vi "Tester by yuval.vi"() -> ()   [LabVIEW 2015]
uses:
  source/controls/Treatment Parameters.ctl
  source/controls/Results.ctl
  <vilib>/vision/Image Controls.llb/IMAQ Image.ctl
  <vilib>/vision/driver/NI_Vision_Acquisition_Software.lvlib
  <resource>/objmgr/imaqdx.rc
  <vilib>/vision/NI_Vision_Development_Module.lvlib
panel:
  out "Image Out":T1
  out "Sclera Score":dbl
  out "Results Out":T2={"Center X"=500, "Center Y"=500, "Radius X"=1, "Radius Y"=1, "Circle Match Score"=0, "Sclera Score"=0.0, "Circle Fit Strength"=0, "Circle Match Threshold"=0}
  in  "Camera Name":refnum<k21> caption="IMAQdx Session"
  in  "Video Modes":i32(listbox)
  in  "Stop":bool
  out "Buffer Number":u32
  out "Frame Rate":dbl(knob) scale=0.0..100.0
  out "adjust limbus time":u32
  out "sclera plane time":u32
  in  "Treatment":T3={"Location"=25.0, "Width"=10.0, "Search"=enum."Lower"}
  out "error out":errorcluster
  out "Output Image":T1(plugin-control)
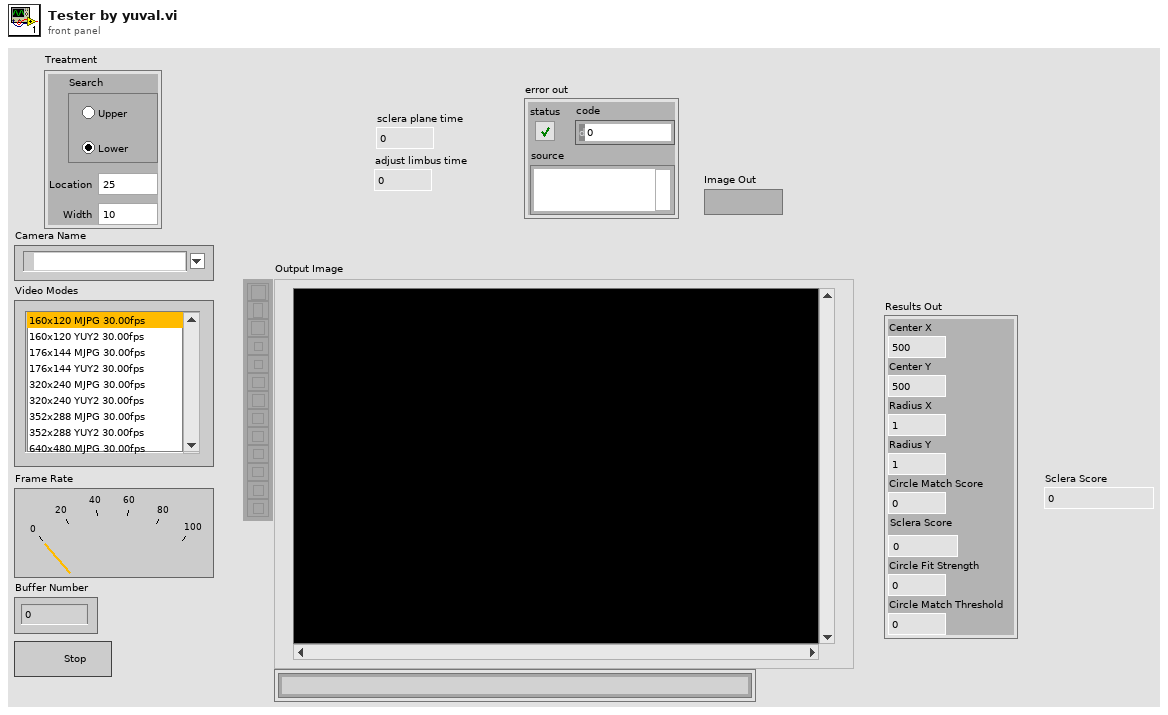
[diagram p1: front panel]
types:
  T1 = typedef "IMAQ Image.ctl" = refnum<image>
  T2 = typedef "Results.ctl" = cluster{"Center X":i32, "Center Y":i32, "Radius X":i32, "Radius Y":i32, "Circle Match Score":i32, "Sclera Score":dbl, "Circle Fit Strength":i32, "Circle Match Threshold":i32}
  T3 = typedef "Treatment Parameters.ctl" = cluster{"Location":dbl, "Width":dbl, "Search":enum32{"Upper", "Lower"}}
  T4 = typedef "IMAQdx.ctl" = refnum<k21>
  T5 = typedef "Images.ctl" = cluster{"Input":T1, "Output":T1, "BufferGray1":T1, "BufferGray2":T1, "TemplatesDown":T1[], "TemplatesUp":T1[], "BufferColor1":T1, "GreenPlane":T1, "ScleraPlane":T1, "RedPlane":T1, "BluePlane":T1}
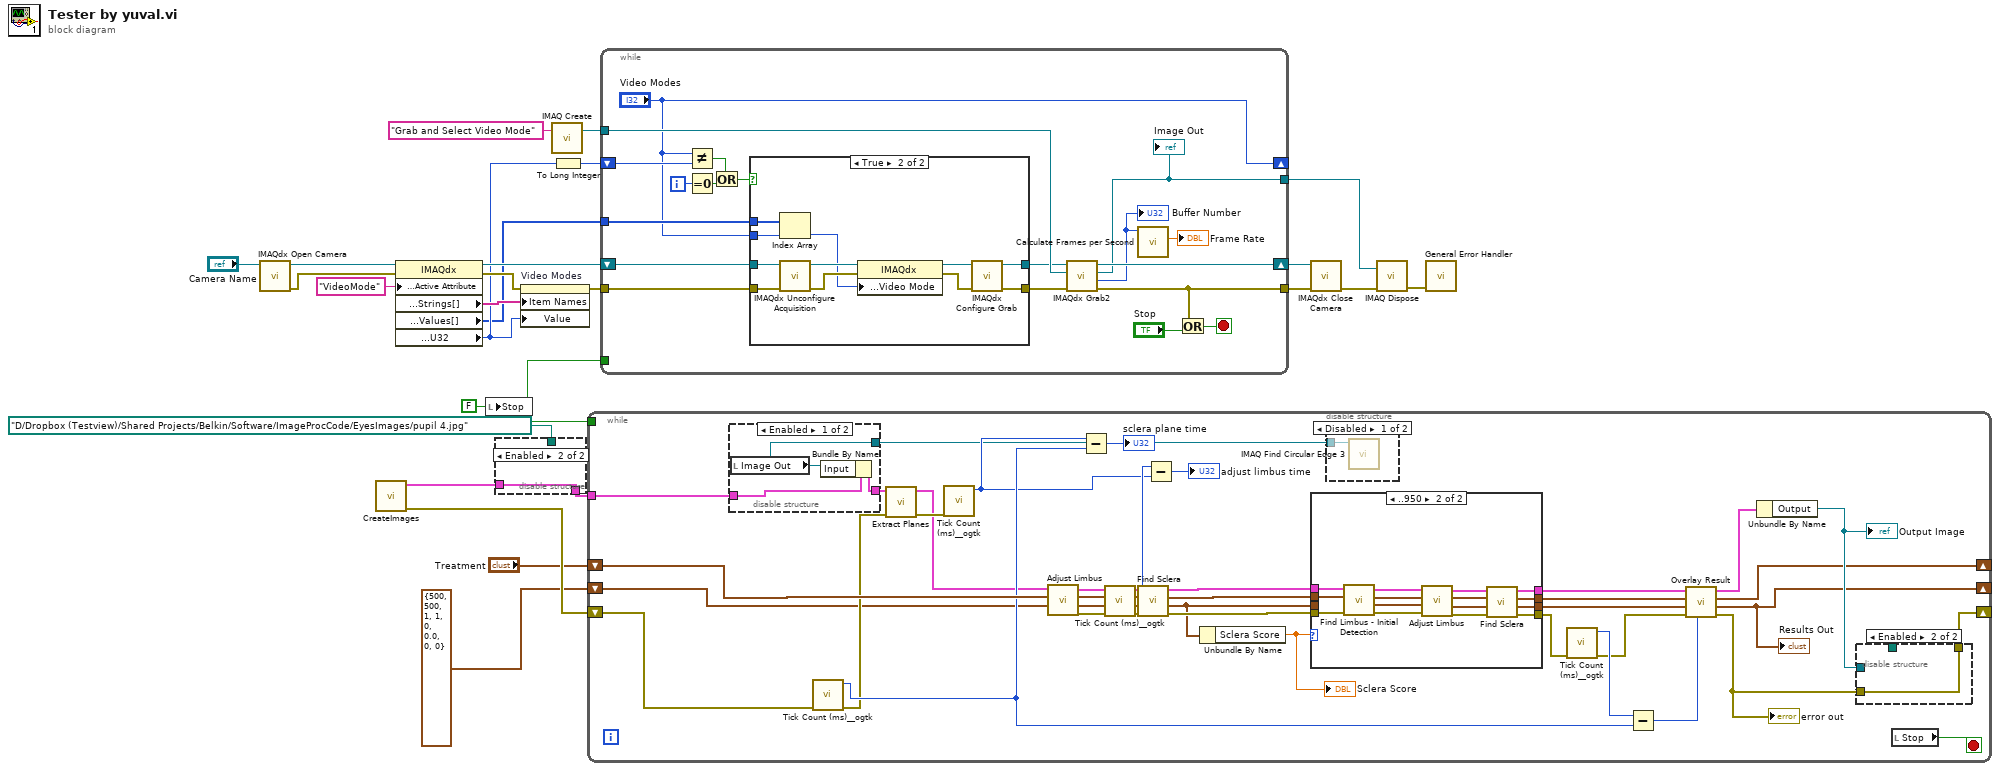
[diagram p0: block diagram]
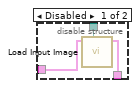
[diagram p2: hidden frame]
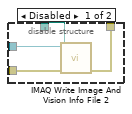
[diagram p5: hidden frame]
diagram:
  w4 = FALSE ("Stop")
  n1 = call <vilib>:"IMAQdx Open Camera.vi"("Session In"="Camera Name") -> ("error out"=w15:errorcluster, "Session Out"=w17:T4)  [unwired: 2 in, 7 out]
  n2 = call "CreateImages.vi"() -> ("error out"=w25:errorcluster, "Images"=w3:T5)  [unwired: 10 in]
  n3 = property class="IMAQdx"(reference=w17, error in=w15, "Camera Attributes:Active Attribute"="VideoMode" ("ActiveAttribute")) -> (reference out=w13:T4, error out=w14:errorcluster, "Camera Attributes:Enum:Strings[]"=w11:string[], "Camera Attributes:Enum:Values[]"=w5:u32[], "Camera Attributes:Value:U32"=w10:u32)
  n4 = local write "Stop"(w4) -> ()
  n5 = disable-structure shown="Enabled" {
    disable-tunnel: w3 -> [w28 w29]
    disable-tunnel: [w27 w29] -> w2
    disable-tunnel: path "D:/Dropbox (Testview)/Shared Projects/Belkin/Software/ImageProcCode/EyesImages/pupil 4.jpg" ("Path") -> [w26 _]
    frame Disabled {
      n6 = call "Load Input Image.vi"("Path"=w26, "Images"=w28) -> ("Images"=w27:T5)  [unwired: 8 in, 1 out]
    }
    frame Enabled {
    }
  }
  n7 = property on="Video Modes" class="LstBox (strict)"(error in=w14, "Item Names"=w11, "Value"=w10) -> (error out=w12:errorcluster)  [unwired: 1 in, 1 out]
  n8 = call "IMAQ Create"("Image Name"="Grab and Select Video Mode") -> ("New Image"=w20:T1)  [unwired: 3 in, 2 out]
  n9 = To Long Integer(number=w10) -> (32bit integer=w9:i32)
  n10 = while {
    tunnel: w2 -> [w33]
    shift-right: [w67] -> _
    shift-left: w25 -> [w31]
    shift-right: [w49] -> _
    shift-left: "Treatment" -> [w50]
    shift-right: [w34] -> _
    shift-left: T2 {"Center X"=500, "Center Y"=500, "Radius X"=1, "Radius Y"=1, "Circle Match Score"=0, "Sclera Score"=0.0, "Circle Fit Strength"=0, "Circle Match Threshold"=0} ("Results Out") -> [w35]
    tunnel: w4 -> [_]
    stop <- w36 stop-if-true
    n11 = disable-structure shown="Enabled" {
      disable-tunnel: w33 -> [w71 w72]
      disable-tunnel: [w70 w72] -> w37
      disable-tunnel: [w69 _] -> w30
      frame Enabled {
        n12 = local read "Image Out"() -> (w69:T1)
        n13 = Bundle By Name(cluster=w71, "Input"=w69) -> (w70:T5)
      }
      frame Disabled {
      }
    }
    n14 = call <userlib>:"Tick Count (ms)__ogtk.vi"("error in (no error)"=w31) -> ("error out"=w40:errorcluster, "millisecond timer value"=w45:u32)  [unwired: 9 in]
    n15 = call "Extract Planes.vi"("error in (no error)"=w40, "Images"=w37) -> ("error out"=w41:errorcluster, "Images"=w39:T5)  [unwired: 8 in]
    n16 = call <userlib>:"Tick Count (ms)__ogtk.vi"("error in (no error)"=w41) -> ("millisecond timer value"=w38:u32)  [unwired: 9 in, 1 out]
    n17 = call "Adjust Limbus.vi"("Results"=w35, "Treatment"=w50, "Images"=w39) -> ("error out"=w55:errorcluster, "Results"=w57:T2, "Treatment"=w56:T3, "Images"=w54:T5)  [unwired: 5 in]
    n18 = Subtract(x=w38, y=w45) -> (x-y=→"sclera plane time":u32)
    n19 = call <userlib>:"Tick Count (ms)__ogtk.vi"("error in (no error)"=w55) -> ("error out"=w46:errorcluster, "millisecond timer value"=w42:u32)  [unwired: 9 in]
    n20 = call "Find Sclera.vi"("error in (no error)"=w46, "Results"=w57, "Treatment"=w56, "Images"=w54) -> ("error out"=w51:errorcluster, "Results"=w47:T2, "Treatment"=w52:T3, "Images"=w53:T5)  [unwired: 4 in]
    n21 = Subtract(x=w42, y=w38) -> (x-y=→"adjust limbus time":u32)
    n22 = Unbundle By Name(w47) -> ("Sclera Score"=w48:dbl)
    "Sclera Score" <- w48
    n23 = case shown="..950" w48 {
      tunnel: [w81 w96] -> w66
      tunnel: [w80 w95] -> w65
      tunnel: [w79 w94] -> w64
      tunnel: [w78 w86] -> w61
      tunnel: w53 -> [w81 w84]
      tunnel: w52 -> [w80 w83]
      tunnel: w51 -> [w78 w82]
      tunnel: w47 -> [w79 _]
      frame 951.. {
      }
      frame ..950 {
        n24 = call "Find Limbus - Initial Detection.vi"("error in (no error)"=w82, "Treatment in"=w83, "Images in"=w84) -> ("error out"=w85:errorcluster, "Results"=w89:T2, "Treatment Out"=w90:T3, "Images out"=w93:T5)  [unwired: 5 in]
        n25 = call "Adjust Limbus.vi"("error in (no error)"=w85, "Results"=w89, "Treatment"=w90, "Images"=w93) -> ("error out"=w91:errorcluster, "Results"=w87:T2, "Treatment"=w88:T3, "Images"=w92:T5)  [unwired: 4 in]
        n26 = call "Find Sclera.vi"("error in (no error)"=w91, "Results"=w87, "Treatment"=w88, "Images"=w92) -> ("error out"=w86:errorcluster, "Results"=w94:T2, "Treatment"=w95:T3, "Images"=w96:T5)  [unwired: 4 in]
      }
    }
    n27 = disable-structure shown="Disabled" {
      disable-tunnel: w30 -> [w68 _]
      frame Disabled {
        n28 = call "IMAQ Find Circular Edge 3"("Image"=w68) -> ()  [unwired: 6 in, 5 out]
      }
      frame Enabled {
      }
    }
    n29 = call <userlib>:"Tick Count (ms)__ogtk.vi"("error in (no error)"=w61) -> ("error out"=w59:errorcluster, "millisecond timer value"=w60:u32)  [unwired: 9 in]
    n30 = Subtract(x=w60, y=w45) -> (x-y=w58:u32)
    n31 = call "Overlay Result.vi"("Processing Time"=w58, "error in (no error)"=w59, "Results"=w64, "Treatment"=w65, "Images"=w66) -> ("error out"=w32:errorcluster, "Results Out"=w34:T2, "Treatment Out"=w49:T3, "Images"=w63:T5)  [unwired: 3 in]
    "Results Out" <- w34
    "error out" <- w32
    n32 = Unbundle By Name(w63) -> ("Output"=w62:T1)
    "Output Image" <- w62
    n33 = disable-structure shown="Enabled" {
      disable-tunnel: _ -> [w76 _]
      disable-tunnel: [w75 w77] -> w67
      disable-tunnel: w62 -> [w74 _]
      disable-tunnel: w32 -> [w73 w77]
      frame Disabled {
        n34 = call "IMAQ Write Image And Vision Info File 2"("error in (no error)"=w73, "File Path"=w76, "Image"=w74) -> ("error out"=w75:errorcluster)  [unwired: 7 in, 1 out]
      }
      frame Enabled {
      }
    }
    n35 = local read "Stop"() -> (w36:bool)
  }
  n36 = while {
    tunnel: w5 -> [w112]
    shift-left: w9 -> [w109]
    shift-right: ["Video Modes"] -> _
    tunnel: w20 -> [w113]
    tunnel: w12 -> [w114]
    tunnel: [w98] -> w22
    shift-right: [w101] -> w19
    shift-left: w13 -> [w115]
    tunnel: [w97] -> w8
    tunnel: w4 -> [_]
    i -> [w105]
    stop <- w110 stop-if-true
    n37 = Not Equal?(x="Video Modes", y=w109) -> (x != y?=w106:bool)
    n38 = Equal To 0?(x=w105) -> (x = 0?=w104:bool)
    n39 = Or(x=w106, y=w104) -> (x .or. y?=w107:bool)
    n40 = case shown="True" w107 {
      tunnel: w115 -> [w117 w126]
      tunnel: w114 -> [w116 w125]
      tunnel: [w117 w122] -> w102
      tunnel: [w116 w123] -> w103
      tunnel: w112 -> [_ w128]
      tunnel: "Video Modes" -> [_ w127]
      frame False {
      }
      frame True {
        n41 = Index Array(array=w128, index=w127) -> (element=w118:u32)
        n42 = call <vilib>:"IMAQdx Unconfigure Acquisition.vi"("error in"=w125, "Session In"=w126) -> ("error out"=w119:errorcluster, "Session Out"=w124:T4)  [unwired: 8 out]
        n43 = property class="IMAQdx"(reference=w124, error in=w119, "Acquisition Attributes:Video Mode"=w118) -> (reference out=w121:T4, error out=w120:errorcluster)
        n44 = call <vilib>:"IMAQdx Configure Grab.vi"("error in"=w120, "Session In"=w121) -> ("error out"=w123:errorcluster, "Session Out"=w122:T4)  [unwired: 1 in, 7 out]
      }
    }
    n45 = call <vilib>:"IMAQdx Grab2.vi"("error in"=w103, "Image In"=w113, "Session In"=w102) -> ("error out"=w98:errorcluster, "Buffer Number Out"=w99:u32, "Image Out"=w97:T1, "Session Out"=w101:T4)  [unwired: 5 in]
    "Buffer Number" <- w99
    "Image Out" <- w97
    n46 = call <vilib>:"Calculate Frames per Second.vi"("Buffer Number"=w99) -> ("Processed Frames/s"=→"Frame Rate":dbl)  [unwired: 8 in, 2 out]
    n47 = Or(x=w98, y="Stop") -> (x .or. y?=w110:bool)
  }
  n48 = call <vilib>:"IMAQdx Close Camera.vi"("error in"=w22, "Session In"=w19) -> ("error out"=w7:errorcluster)  [unwired: 9 out]
  n49 = call "IMAQ Dispose"("Image"=w8, "error in (no error)"=w7) -> ("error out"=w6:errorcluster)  [unwired: 4 in]
  n50 = call <vilib>:"General Error Handler.vi"("error in (no error)"=w6) -> ()  [unwired: 2 in, 13 out]
